vi "TEST-02.vi"() -> ()   [LabVIEW 2017]
panel:
  out "DEC VALUE":i16
  in  "stop":bool
  in  "Bit 0":bool
  in  "Bit 1":bool
  out "Bit 0":bool
  out "Bit 1":bool
  out "Bit 2":bool
  in  "Bit 2":bool
  out "Bit 3":bool
  in  "Bit 3":bool
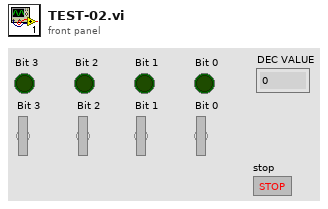
[diagram p1: front panel]
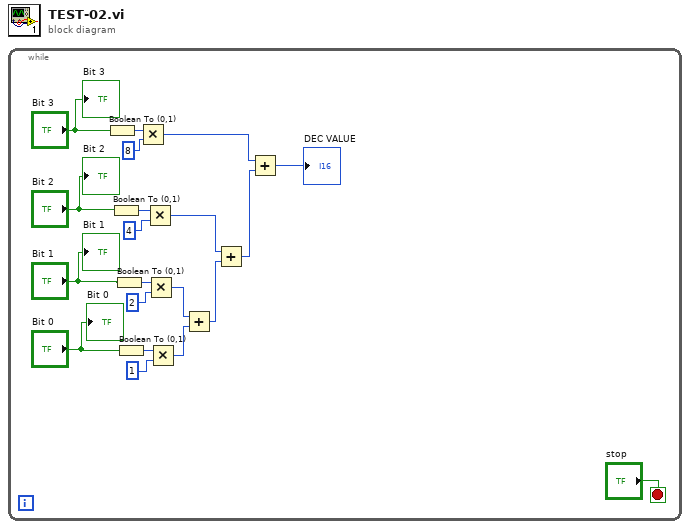
[diagram p0: block diagram]
diagram:
  n1 = while {
    stop <- "stop" stop-if-true
    n2 = Boolean To (0,1)(Boolean="Bit 3") -> (0, 1=w9:i16)
    n3 = Boolean To (0,1)(Boolean="Bit 2") -> (0, 1=w11:i16)
    n4 = Boolean To (0,1)(Boolean="Bit 1") -> (0, 1=w13:i16)
    n5 = Boolean To (0,1)(Boolean="Bit 0") -> (0, 1=w15:i16)
    n6 = Multiply(x=w9, y=i16 8) -> (x*y=w3:i16)
    n7 = Multiply(x=w11, y=i16 4) -> (x*y=w5:i16)
    n8 = Multiply(x=w13, y=i16 2) -> (x*y=w7:i16)
    n9 = Multiply(x=w15, y=i16 1) -> (x*y=w6:i16)
    n10 = Add(x=w7, y=w6) -> (x+y=w4:i16)
    n11 = Add(x=w5, y=w4) -> (x+y=w2:i16)
    n12 = Add(x=w3, y=w2) -> (x+y=→"DEC VALUE":i16)
    "Bit 3" <- "Bit 3"
    "Bit 2" <- "Bit 2"
    "Bit 1" <- "Bit 1"
    "Bit 0" <- "Bit 0"
  }
